vi "Configure Module.vi"(8 "error in (no error)":errorcluster, 10 "IOV ref in":variant, 11 "Module Template in":refnum<class "9219.lvclass">) -> (0 "error out":errorcluster, 2 "IOV ref out":variant, 3 "Module Template out":refnum<class "9219.lvclass">)   [LabVIEW 2019, in "Modules.lvlib" / "9219.lvclass"]
uses:
  9219.lvclass
  <resource>/objmgr/cRIO.rc
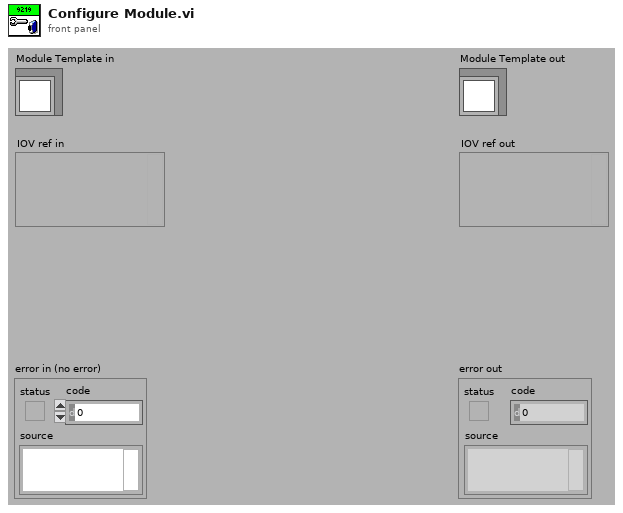
[diagram p1: front panel]
types:
  T1 = cluster{"Degree range":u32, "Digital threshold":dbl, "Range / Mode":u32, "RTD type":u32, "RTD A":dbl, "RTD B":dbl, "RTD C":dbl, "RTD Ro":dbl, "Thermocouple type":u32}[]
  T2 = cluster{"Degree range":u32, "Digital threshold":dbl, "Range / Mode":u32, "RTD type":u32, "RTD A":dbl, "RTD B":dbl, "RTD C":dbl, "RTD Ro":dbl, "Thermocouple type":u32}
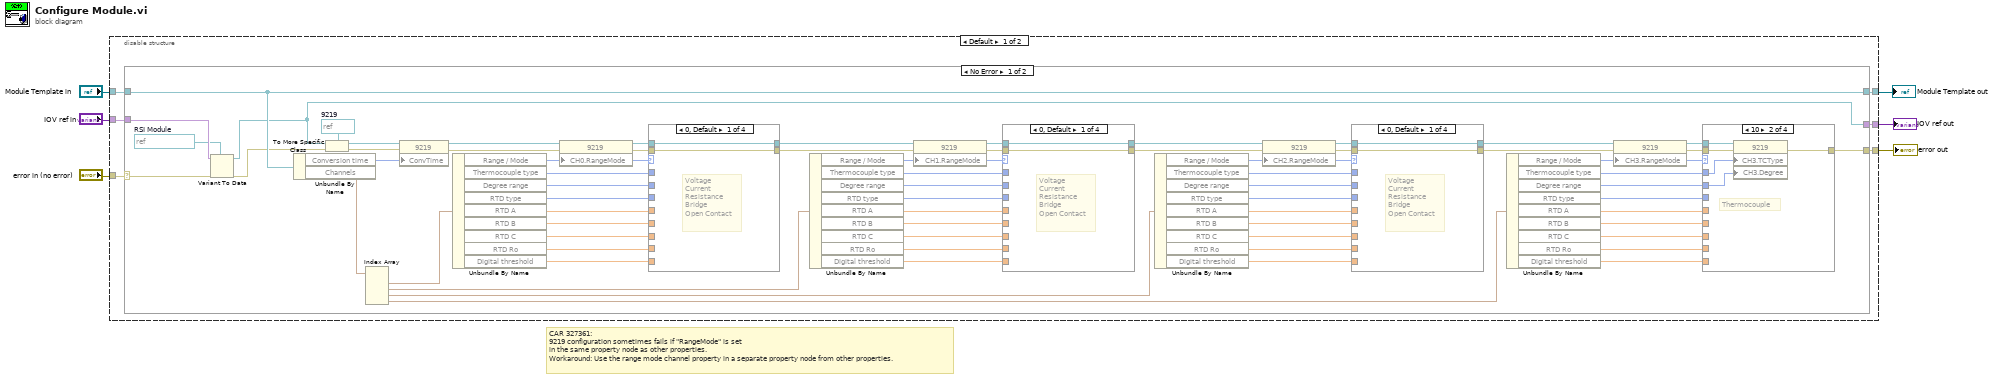
[diagram p0: block diagram]
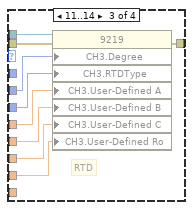
[diagram p3: hidden frame]
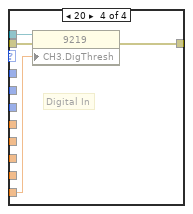
[diagram p4: hidden frame]
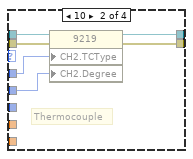
[diagram p5: hidden frame]
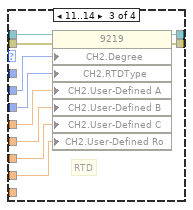
[diagram p6: hidden frame]
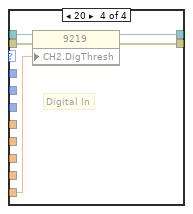
[diagram p7: hidden frame]
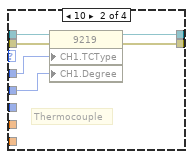
[diagram p8: hidden frame]
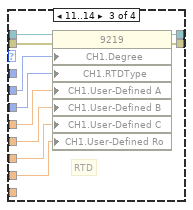
[diagram p9: hidden frame]
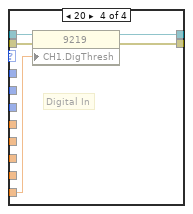
[diagram p10: hidden frame]
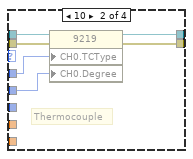
[diagram p11: hidden frame]
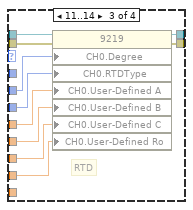
[diagram p12: hidden frame]
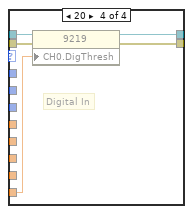
[diagram p13: hidden frame]
diagram:
  # "CAR 327361:\n9219 configuration sometimes fails if \"RangeMode\" is set\nin the same property node as other properties. \nWorkaround: Use the range mode channel property in a separate property node from other properties."
  n1 = disable-structure shown="Default" {
    disable-tunnel: "error in (no error)" -> [w12 w172]
    disable-tunnel: [w11 w172] -> w5
    disable-tunnel: "Module Template in" -> [w10 w174]
    disable-tunnel: [w9 w174] -> w3
    disable-tunnel: "IOV ref in" -> [w8 w173]
    disable-tunnel: [w7 w173] -> w1
    frame condition #0 {
      n2 = case shown="No Error" w12 {
        selector: w12 -> [w79 w171]
        tunnel: [w17 w171] -> w11
        tunnel: [w80 w170] -> w9
        tunnel: w10 -> [w80 w170]
        tunnel: w8 -> [w15 w169]
        tunnel: [w14 w169] -> w7
        frame No Error {
          w13 = refnum<k21> refnum  # RSI Module
          w78 = refnum<k21> refnum  # 9219
          n3 = Variant To Data(error in=w79, type=w13, Variant=w15) -> (data=w14:refnum<k21>, error out=w16:errorcluster)
          n4 = Unbundle By Name(w80) -> ("Conversion time"=w75:u32, "Channels"=w74:T1)
          n5 = To More Specific Class(target class=w78, reference=w14, error in=w16) -> (specific class reference=w77:refnum<k21>, error out=w76:errorcluster)
          n6 = Index Array(array=w74) -> (element #1=w62:T2, element #2=w63:T2, element #3=w64:T2, element #4=w65:T2)  [unwired: 4 in]
          n7 = property class="9219"(reference=w77, error in=w76, "ConvTime"=w75) -> (reference out=w60:refnum<k21>, error out=w57:errorcluster)
          n8 = Unbundle By Name(w62) -> ("Range / Mode"=w61:u32, "Thermocouple type"=w66:u32, "Degree range"=w67:u32, "RTD type"=w68:u32, "RTD A"=w69:dbl, "RTD B"=w70:dbl, "RTD C"=w71:dbl, "RTD Ro"=w72:dbl, "Digital threshold"=w73:dbl)
          n9 = property class="9219"(reference=w60, error in=w57, "CH0.RangeMode"=w61) -> (reference out=w59:refnum<k21>, error out=w58:errorcluster)
          n10 = case shown="0, Default" w61 {
            tunnel: w66 -> [_ w153 _ _]
            tunnel: w67 -> [_ w152 w163 _]
            tunnel: w68 -> [_ _ w158 _]
            tunnel: w69 -> [_ _ w159 _]
            tunnel: w70 -> [_ _ w160 _]
            tunnel: w71 -> [_ _ w161 _]
            tunnel: w72 -> [_ _ w162 _]
            tunnel: w73 -> [_ _ _ w168]
            tunnel: w59 -> [w147 w149 w157 w167]
            tunnel: w58 -> [w146 w148 w156 w166]
            tunnel: [w147 w151 w155 w165] -> w54
            tunnel: [w146 w150 w154 w164] -> w52
            frame 0, Default {
              # "Voltage\nCurrent\nResistance\nBridge\nOpen Contact"
            }
            frame 10 {
              # "Thermocouple"
              n11 = property class="9219"(reference=w149, error in=w148, "CH0.TCType"=w153, "CH0.Degree"=w152) -> (reference out=w151:refnum<k21>, error out=w150:errorcluster)
            }
            frame 11..14 {
              # "RTD"
              n12 = property class="9219"(reference=w157, error in=w156, "CH0.Degree"=w163, "CH0.RTDType"=w158, "CH0.User-Defined A"=w159, "CH0.User-Defined B"=w160, "CH0.User-Defined C"=w161, "CH0.User-Defined Ro"=w162) -> (reference out=w155:refnum<k21>, error out=w154:errorcluster)
            }
            frame 20 {
              # "Digital In"
              n13 = property class="9219"(reference=w167, error in=w166, "CH0.DigThresh"=w168) -> (reference out=w165:refnum<k21>, error out=w164:errorcluster)
            }
          }
          n14 = Unbundle By Name(w63) -> ("Range / Mode"=w53:u32, "Thermocouple type"=w51:u32, "Degree range"=w50:u32, "RTD type"=w49:u32, "RTD A"=w48:dbl, "RTD B"=w47:dbl, "RTD C"=w46:dbl, "RTD Ro"=w45:dbl, "Digital threshold"=w44:dbl)
          n15 = property class="9219"(reference=w54, error in=w52, "CH1.RangeMode"=w53) -> (reference out=w56:refnum<k21>, error out=w55:errorcluster)
          n16 = case shown="0, Default" w53 {
            tunnel: w51 -> [_ w130 _ _]
            tunnel: w50 -> [_ w129 w140 _]
            tunnel: w49 -> [_ _ w135 _]
            tunnel: w48 -> [_ _ w136 _]
            tunnel: w47 -> [_ _ w137 _]
            tunnel: w46 -> [_ _ w138 _]
            tunnel: w45 -> [_ _ w139 _]
            tunnel: w44 -> [_ _ _ w145]
            tunnel: w56 -> [w124 w126 w134 w144]
            tunnel: w55 -> [w123 w125 w133 w143]
            tunnel: [w124 w128 w132 w142] -> w41
            tunnel: [w123 w127 w131 w141] -> w40
            frame 0, Default {
              # "Voltage\nCurrent\nResistance\nBridge\nOpen Contact"
            }
            frame 10 {
              # "Thermocouple"
              n17 = property class="9219"(reference=w126, error in=w125, "CH1.TCType"=w130, "CH1.Degree"=w129) -> (reference out=w128:refnum<k21>, error out=w127:errorcluster)
            }
            frame 11..14 {
              # "RTD"
              n18 = property class="9219"(reference=w134, error in=w133, "CH1.Degree"=w140, "CH1.RTDType"=w135, "CH1.User-Defined A"=w136, "CH1.User-Defined B"=w137, "CH1.User-Defined C"=w138, "CH1.User-Defined Ro"=w139) -> (reference out=w132:refnum<k21>, error out=w131:errorcluster)
            }
            frame 20 {
              # "Digital In"
              n19 = property class="9219"(reference=w144, error in=w143, "CH1.DigThresh"=w145) -> (reference out=w142:refnum<k21>, error out=w141:errorcluster)
            }
          }
          n20 = Unbundle By Name(w64) -> ("Range / Mode"=w39:u32, "Thermocouple type"=w38:u32, "Degree range"=w37:u32, "RTD type"=w36:u32, "RTD A"=w35:dbl, "RTD B"=w34:dbl, "RTD C"=w33:dbl, "RTD Ro"=w32:dbl, "Digital threshold"=w31:dbl)
          n21 = property class="9219"(reference=w41, error in=w40, "CH2.RangeMode"=w39) -> (reference out=w42:refnum<k21>, error out=w43:errorcluster)
          n22 = case shown="0, Default" w39 {
            tunnel: w38 -> [_ w107 _ _]
            tunnel: w37 -> [_ w106 w117 _]
            tunnel: w36 -> [_ _ w112 _]
            tunnel: w35 -> [_ _ w113 _]
            tunnel: w34 -> [_ _ w114 _]
            tunnel: w33 -> [_ _ w115 _]
            tunnel: w32 -> [_ _ w116 _]
            tunnel: w31 -> [_ _ _ w122]
            tunnel: w42 -> [w101 w103 w111 w121]
            tunnel: w43 -> [w100 w102 w110 w120]
            tunnel: [w101 w105 w109 w119] -> w28
            tunnel: [w100 w104 w108 w118] -> w27
            frame 0, Default {
              # "Voltage\nCurrent\nResistance\nBridge\nOpen Contact"
            }
            frame 10 {
              # "Thermocouple"
              n23 = property class="9219"(reference=w103, error in=w102, "CH2.TCType"=w107, "CH2.Degree"=w106) -> (reference out=w105:refnum<k21>, error out=w104:errorcluster)
            }
            frame 11..14 {
              # "RTD"
              n24 = property class="9219"(reference=w111, error in=w110, "CH2.Degree"=w117, "CH2.RTDType"=w112, "CH2.User-Defined A"=w113, "CH2.User-Defined B"=w114, "CH2.User-Defined C"=w115, "CH2.User-Defined Ro"=w116) -> (reference out=w109:refnum<k21>, error out=w108:errorcluster)
            }
            frame 20 {
              # "Digital In"
              n25 = property class="9219"(reference=w121, error in=w120, "CH2.DigThresh"=w122) -> (reference out=w119:refnum<k21>, error out=w118:errorcluster)
            }
          }
          n26 = Unbundle By Name(w65) -> ("Range / Mode"=w26:u32, "Thermocouple type"=w25:u32, "Degree range"=w24:u32, "RTD type"=w23:u32, "RTD A"=w22:dbl, "RTD B"=w21:dbl, "RTD C"=w20:dbl, "RTD Ro"=w19:dbl, "Digital threshold"=w18:dbl)
          n27 = property class="9219"(reference=w28, error in=w27, "CH3.RangeMode"=w26) -> (reference out=w30:refnum<k21>, error out=w29:errorcluster)
          n28 = case shown="10" w26 {
            tunnel: w25 -> [_ w86 _ _]
            tunnel: w24 -> [_ w85 w95 _]
            tunnel: w23 -> [_ _ w90 _]
            tunnel: w22 -> [_ _ w91 _]
            tunnel: w21 -> [_ _ w92 _]
            tunnel: w20 -> [_ _ w93 _]
            tunnel: w19 -> [_ _ w94 _]
            tunnel: w18 -> [_ _ _ w99]
            tunnel: w30 -> [_ w83 w89 w98]
            tunnel: w29 -> [w81 w82 w88 w97]
            tunnel: [w81 w84 w87 w96] -> w17
            frame 0, Default {
              # "Voltage\nCurrent\nResistance\nBridge\nOpen Contact"
            }
            frame 10 {
              # "Thermocouple"
              n29 = property class="9219"(reference=w83, error in=w82, "CH3.TCType"=w86, "CH3.Degree"=w85) -> (error out=w84:errorcluster)  [unwired: 1 out]
            }
            frame 11..14 {
              # "RTD"
              n30 = property class="9219"(reference=w89, error in=w88, "CH3.Degree"=w95, "CH3.RTDType"=w90, "CH3.User-Defined A"=w91, "CH3.User-Defined B"=w92, "CH3.User-Defined C"=w93, "CH3.User-Defined Ro"=w94) -> (error out=w87:errorcluster)  [unwired: 1 out]
            }
            frame 20 {
              # "Digital In"
              n31 = property class="9219"(reference=w98, error in=w97, "CH3.DigThresh"=w99) -> (error out=w96:errorcluster)  [unwired: 1 out]
            }
          }
        }
        frame Error {
        }
      }
    }
    frame condition #1 (active) {
    }
  }
  "error out" <- w5
  "Module Template out" <- w3
  "IOV ref out" <- w1
